vi "Corr Digitizer Open.vi"(8 "error in":errorcluster, 11 "digitizer corrections in":T1) -> (0 "error out":errorcluster, 1 "all channels of the correction valid?":bool, 2 "some correction selected?":bool, 3 "digitizer corrections out":T1)   [LabVIEW 2013]
doc: "This VI will invoke open dialog for digitizer correction selection. If selected it will load it and check if it is valid."
uses:
  Corr Digitizers.ctl
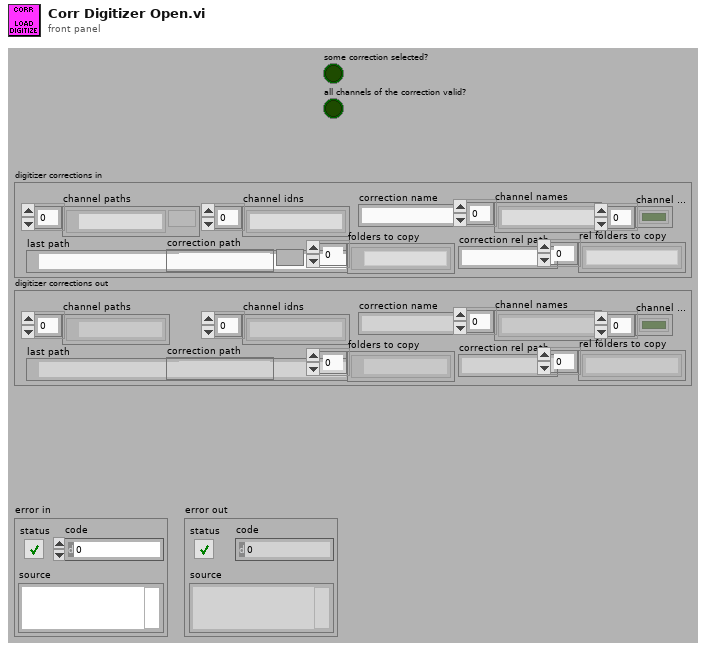
[diagram p1: front panel]
types:
  T1 = typedef "Corr Digitizers.ctl" = cluster{"last path":path, "channel paths":path[], "channel idns":string[], "correction name":string, "channel names":string[], "folders to copy":path[], "channel valid":bool[], "correction path":path, "correction rel path":string, "rel folders to copy":string[]}
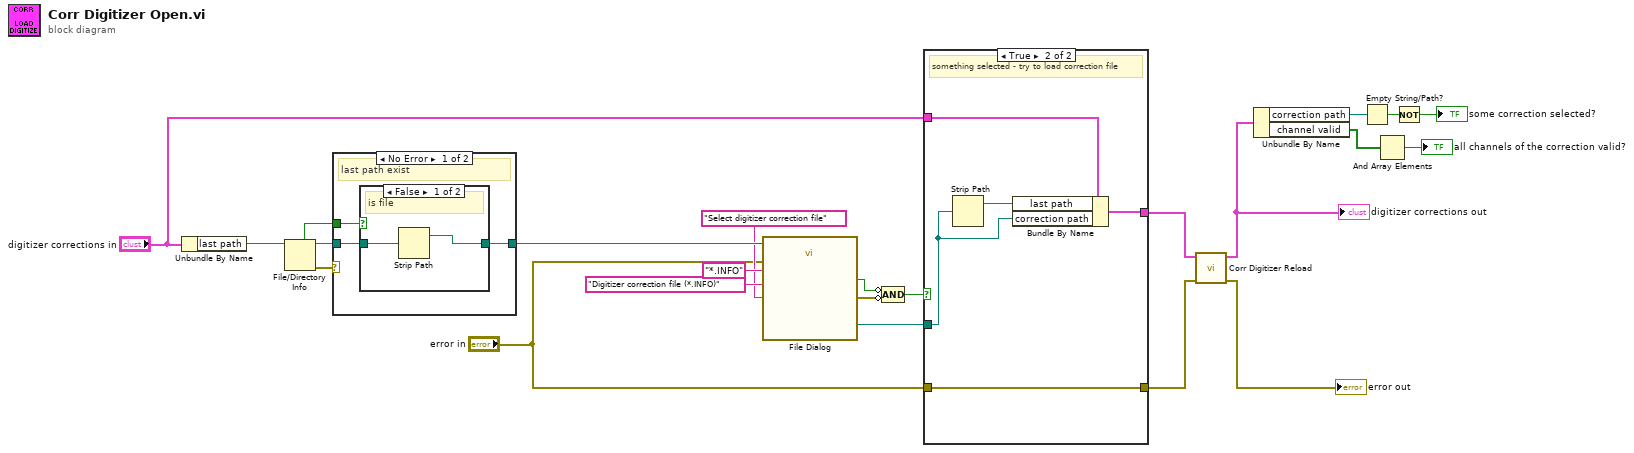
[diagram p0: block diagram]
diagram:
  n1 = Unbundle By Name("digitizer corrections in") -> ("last path"=w23:path)
  n2 = File/Directory Info(path=w23) -> (path out=w21:path, directory=w20:bool, error out=w22:errorcluster)  [unwired: 1 in, 4 out]
  n3 = case shown="No Error" w22 {
    tunnel: w21 -> [w25 w30]
    tunnel: w20 -> [w26 _]
    tunnel: [w24 w30] -> w19
    frame No Error {
      # "last path exist"
      n4 = case shown="False" w26 {
        tunnel: w25 -> [w28 w29]
        tunnel: [w27 w29] -> w24
        frame False {
          # "is file"
          n5 = Strip Path(path=w28) -> (stripped path=w27:path)  [unwired: 1 out]
        }
        frame True {
          # "is folder"
        }
      }
    }
    frame Error {
    }
  }
  n6 = call "File Dialog"("start path"=w19, "prompt"="Select digitizer correction file", "error in"="error in", "pattern (all files)"="*.INFO", "pattern label"="Digitizer correction file (*.INFO)") -> ("selected path"=w12:path, "cancelled"=w15:bool, "error out"=w13:errorcluster)  [unwired: 7 in, 1 out]
  n7 = Compound Arithmetic op=AND(invert w15, invert w13) -> (w14:bool)
  n8 = case shown="True" w14 {
    tunnel: w12 -> [_ w35]
    tunnel: "error in" -> [w32 w34]
    tunnel: [w32 w34] -> w8
    tunnel: "digitizer corrections in" -> [w31 w37]
    tunnel: [w31 w33] -> w9
    frame False {
    }
    frame True {
      # "something selected - try to load correction file"
      n9 = Strip Path(path=w35) -> (stripped path=w36:path)  [unwired: 1 out]
      n10 = Bundle By Name(cluster=w37, "last path"=w36, "correction path"=w35) -> (w33:T1)
    }
  }
  n11 = call "Corr Digitizer Reload.vi"("error in (no error)"=w8, "digitizer corrections in"=w9) -> ("error out"=→"error out":errorcluster, "digitizer corrections out"=w6:T1)  [unwired: 8 in]
  "digitizer corrections out" <- w6
  n12 = Unbundle By Name(w6) -> ("correction path"=w5:path, "channel valid"=w4:bool[])
  n13 = Empty String/Path?(string/path=w5) -> (empty?=w3:bool)
  n14 = And Array Elements(Boolean array=w4) -> (logical AND=→"all channels of the correction valid?":bool)
  n15 = Not(x=w3) -> (.not. x?=→"some correction selected?":bool)
